vi "Customers_Create.vi"(0 "reference in":refnum<class "Customers.lvclass">, 1 "Group":string, 5 "error in (no error)":errorcluster) -> (14 "reference out":refnum<class "Customers.lvclass">, 19 "error out":errorcluster)   [LabVIEW 2020, in "Customers.lvclass"]
uses:
  Customers.lvclass
  C:/Projects/OpenGDS_DesignPatterns/Bridge1/CustomersBase_class/CustomersBase.lvclass
  CustomersBase_class/CustomersBase.lvclass
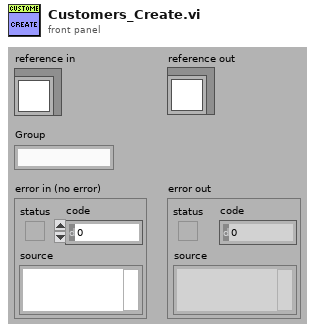
[diagram p1: front panel]
types:
  T1 = typedef "Customers.lvclass/ObjectAttributes.ctl" = cluster{"None":bool}
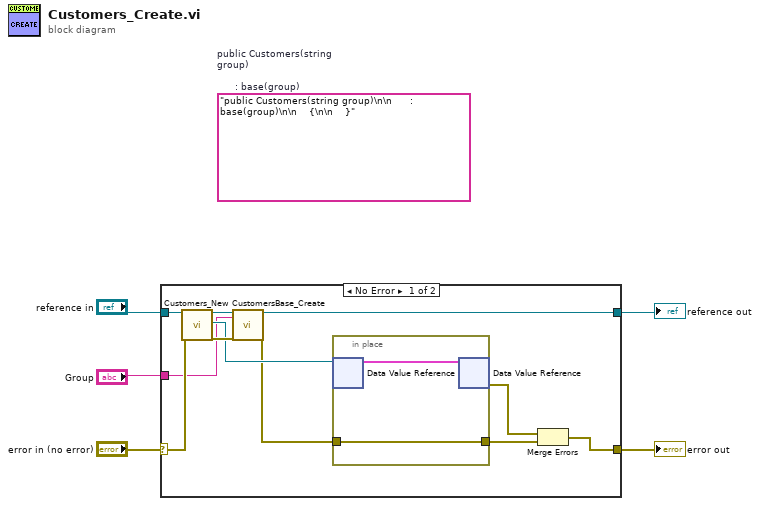
[diagram p0: block diagram]
diagram:
  (unwired) "public Customers(string group)\n\n      : base(group)\n\n    {\n\n    }"  # public Customers(string group)        : base(group)      {      }
  n1 = case shown="No Error" "error in (no error)" {
    selector: "error in (no error)" -> [w15 w20]
    tunnel: [w13 w20] -> w4
    tunnel: "reference in" -> [w16 w19]
    tunnel: [w10 w19] -> w2
    tunnel: "Group" -> [w6 _]
    frame No Error {
      n2 = call "Customers_New.vi"("reference in"=w16, "error in (no error)"=w15) -> ("reference out"=w12:refnum<class "Customers.lvclass">, "DVRRefOut"=w9:refnum<data-value>, "error out"=w11:errorcluster)  [unwired: 14 in, 1 out]
      n3 = call "CustomersBase_Create.vi"("reference in"=w12, "Group"=w6, "error in (no error)"=w11) -> ("reference out"=w10:refnum<class "Customers.lvclass">, "error out"=w8:errorcluster)  [unwired: 15 in]
      n4 = in-place {
        in-place-border: w8 -> [w18]
        in-place-border: [w18] -> w7
        n5 = in-place-dvr #1(w9) -> (w17:T1)  [unwired: 1 out]
        n6 = in-place-dvr #1(w17) -> (w14:errorcluster)  [unwired: 1 out]
      }
      n7 = Merge Errors(w14, w7) -> (w13:errorcluster)
    }
    frame Error {
    }
  }
  "error out" <- w4
  "reference out" <- w2
